vi "BRig_dataMTrig_Solenoid_Td.vi"() -> (2 "output_Solenoid_Td":i32)   [LabVIEW 2014]
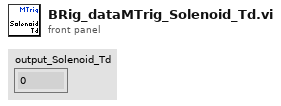
[diagram p1: front panel]
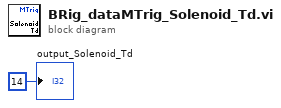
[diagram p0: block diagram]
diagram:
  "output_Solenoid_Td" <- 14 ("output_iBlock")
